vi "SIM RK Variable Coefficients.vi"(1 "continuous integrator":T2=enum."RK 45") -> (0 "Runga-Kutte data":T1={"weighting coefficients"=[[0.2, 0.0, 0.0, 0.0, 0.0, 0.0], [0.075, 0.225, 0.0, 0.0, 0.0, 0.0], [0.9777777777777777, -3.7333333333333334, 3.5555555555555554, 0.0, 0.0, 0.0], [2.9525986892242035, -11.595793324188385, 9.822892851699436, -0.2908093278463649, 0.0, 0.0], [2.8462752525252526, -10.757575757575758, 8.906422717743473, 0.2784090909090909, -0.2735313036020583, 0.0], [0.09114583333333333, 0.0, 0.44923629829290207, 0.6510416666666666, -0.322376179245283, 0.13095238095238096]], "time step fractions"=[0.2, 0.3, 0.8, 0.8888888888888888, 1.0, 1.0], "Number of sub steps"=6, "error coefficients"=[0.09114583333333333, 0.0, 0.44923629829290207, 0.6510416666666666, -0.322376179245283, 0.13095238095238096, 0.0], "error order"=5} {"error coefficients" format="%.5f"; "time step fractions" format="%.5f"; "weighting coefficients" format="%.5f"})   [LabVIEW 2014]
uses:
  SIM integration method.ctl
  SIM Runga-Kutte data - variable step.ctl
panel:
  in  "Runga-Kutte data - Shampine Bogacki 3(2)":T1={"weighting coefficients"=[[0.5, 0.0, 0.0], [0.0, 0.75, 0.0], [0.2222222222222222, 0.3333333333333333, 0.4444444444444444]], "time step fractions"=[0.5, 0.75, 1.0], "Number of sub steps"=3, "error coefficients"=[-0.06944444444444448, 0.08333333333333331, 0.1111111111111111, -0.125], "error order"=3} {"error coefficients" format="%.5f"; "time step fractions" format="%.5f"; "weighting coefficients" format="%.5f"}
  in  "Runga-Kutte data - Dormand Prince 5(4)":T1={"weighting coefficients"=[[0.2, 0.0, 0.0, 0.0, 0.0, 0.0], [0.075, 0.225, 0.0, 0.0, 0.0, 0.0], [0.9777777777777777, -3.7333333333333334, 3.5555555555555554, 0.0, 0.0, 0.0], [2.9525986892242035, -11.595793324188385, 9.822892851699436, -0.2908093278463649, 0.0, 0.0], [2.8462752525252526, -10.757575757575758, 8.906422717743473, 0.2784090909090909, -0.2735313036020583, 0.0], [0.09114583333333333, 0.0, 0.44923629829290207, 0.6510416666666666, -0.322376179245283, 0.13095238095238096]], "time step fractions"=[0.2, 0.3, 0.8, 0.8888888888888888, 1.0, 1.0], "Number of sub steps"=6, "error coefficients"=[0.0012326388888888873, 0.0, -0.004252770290506136, 0.036979166666666674, -0.05086379716981132, 0.04190476190476192, -0.025], "error order"=5} {"error coefficients" format="%.5f"; "time step fractions" format="%.5f"; "weighting coefficients" format="%.5f"}
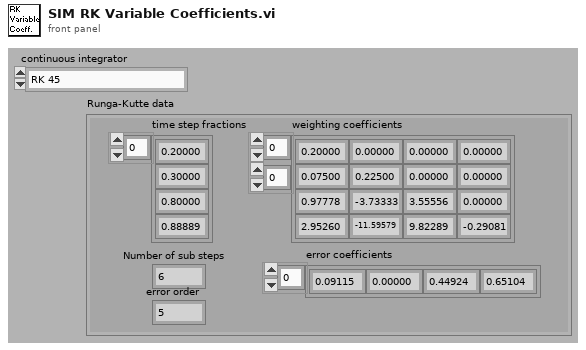
[diagram p1: front panel]
types:
  T1 = typedef "SIM Runga-Kutte data - variable step.ctl" = cluster{"weighting coefficients":dbl[][], "time step fractions":dbl[], "Number of sub steps":i32, "error coefficients":dbl[], "error order":i32}
  T2 = typedef "SIM integration method.ctl" = enum16{"RK 1 (Euler)", "Linearizer", "State Query", "Trim Eval", "Adams", "RK 3", "RK 4", "RK 45", "BDF", "RK 2", "RK 23", "Rosenbrock", "Discrete States Only"}
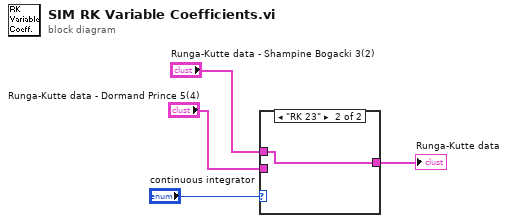
[diagram p0: block diagram]
diagram:
  n1 = case shown="\"RK 23\"" "continuous integrator" {
    tunnel: "Runga-Kutte data - Dormand Prince 5(4)" -> [w5 _]
    tunnel: "Runga-Kutte data - Shampine Bogacki 3(2)" -> [_ w6]
    tunnel: [w5 w6] -> w1
    frame "RK 45", Default {
    }
    frame "RK 23" {
    }
  }
  "Runga-Kutte data" <- w1
